vi "ClusterRef to Label-Value-Arrays.vi"(8 "error in (no error)":errorcluster, 11 "Cluster in":refnum<vi>) -> (0 "error out":errorcluster, 3 "Labels-Values Cluster":cluster{string[], variant[]})   [LabVIEW 2023, in "Message Queue Helper.lvlib"]
uses:
  Message Queue Helper.lvlib
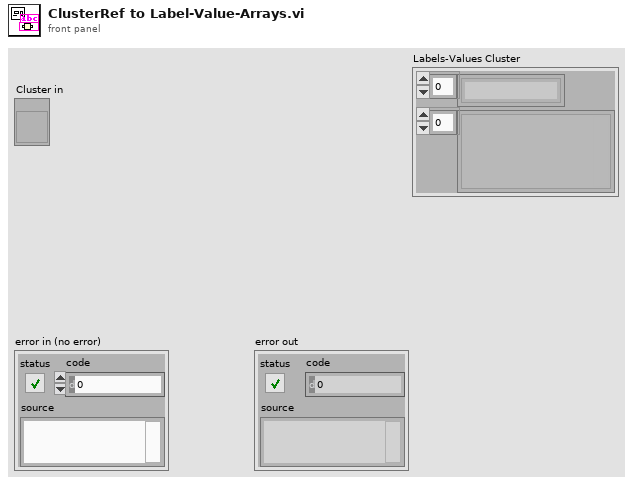
[diagram p1: front panel]
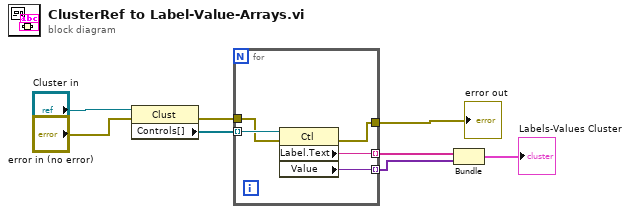
[diagram p0: block diagram]
diagram:
  n1 = property class="Clust"(reference="Cluster in", error in="error in (no error)") -> (error out=w7:errorcluster, "Controls[]"=w6:refnum<vi>[])  [unwired: 1 out]
  n2 = for {
    tunnel: w6 -> [w13] mode=indexing
    tunnel: w7 -> [w12]
    tunnel: [w11] -> w3 mode=indexing
    tunnel: [w10] -> w2 mode=indexing
    tunnel: [w9] -> w8
    n3 = property class="Ctl"(reference=w13, error in=w12) -> (error out=w9:errorcluster, "Label.Text"=w11:string, "Value"=w10:variant)  [unwired: 1 out]
  }
  "error out" <- w8
  n4 = Bundle(w3, w2) -> (→"Labels-Values Cluster":cluster{string[], variant[]})  [unwired: 1 in]
